vi "Upload.vi"(8 "INO":path, 9 "CLI":path, 11 "Selector":string(combo)) -> (3 "concatenated string":string)   [LabVIEW 2025]
uses:
  <vilib>/Utility/error.llb/Trim Whitespace One-Sided.vi
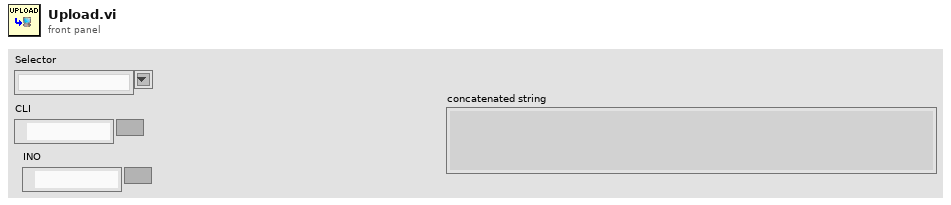
[diagram p1: front panel]
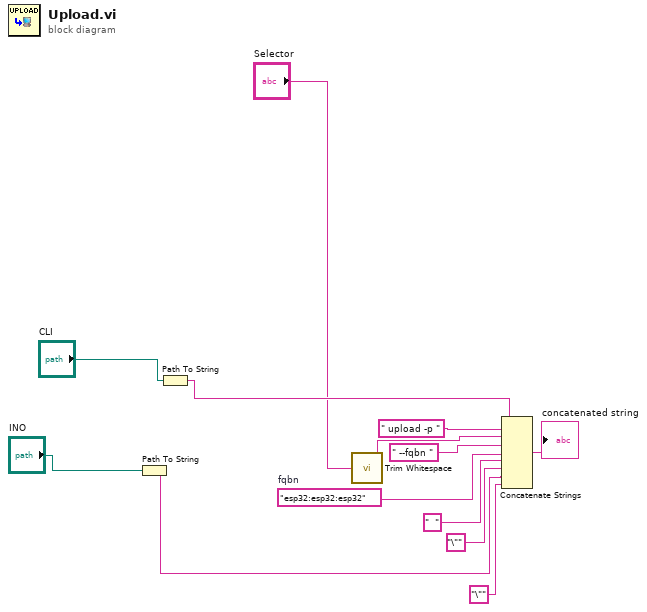
[diagram p0: block diagram]
diagram:
  w7 = "esp32:esp32:esp32"  # fqbn
  n1 = Path To String(path="INO") -> (string=w3:string)
  n2 = Path To String(path="CLI") -> (string=w12:string)
  n3 = call <vilib>:"Trim Whitespace.vi"("string"="Selector") -> ("trimmed string"=w10:string)  [unwired: 1 in]
  n4 = Concatenate Strings(w12, " upload -p " ("string"), w10, " --fqbn " ("string"), w7, "  " ("string"), "\"" ("string"), w3, "\"" ("string")) -> (→"concatenated string":string)
